vi "Establish connection.vi"(8 "error in (no error)":errorcluster, 11 "TCP Writer in":refnum<class "TCP Writer.lvclass">) -> (0 "error out":errorcluster, 3 "output cluster":refnum<class "TCP Writer.lvclass">)   [LabVIEW 2026, in "TALOS.lvlib" / "TCP Writer.lvlib" / "TCP Writer.lvclass"]
uses:
  TCP Writer.lvclass
  TCP Writer.lvclass/TCP Writer.ctl
  Support VIs/Global Constants.vi
  TALOS.lvlib
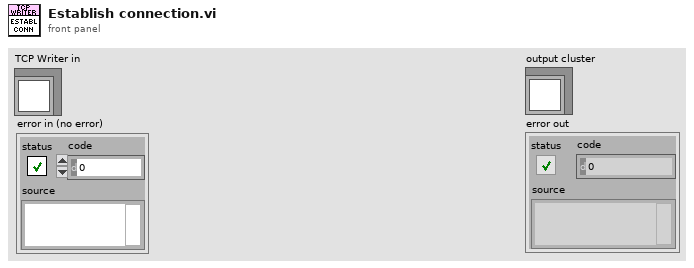
[diagram p1: front panel]
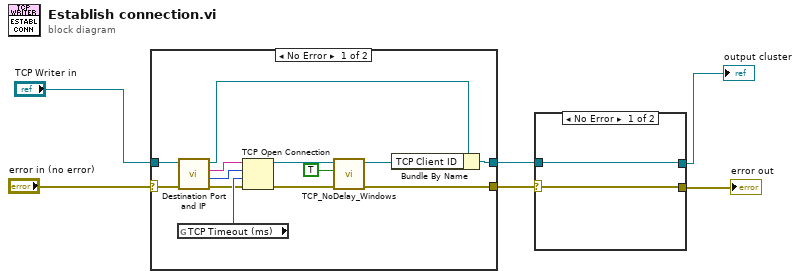
[diagram p0: block diagram]
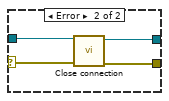
[diagram p3: hidden frame]
diagram:
  n1 = case shown="No Error" "error in (no error)" {
    selector: "error in (no error)" -> [w12 w20]
    tunnel: "TCP Writer in" -> [w14 w21]
    tunnel: [w8 w20] -> w4
    tunnel: [w7 w21] -> w3
    frame No Error {
      n2 = global read "Global Constants.vi" "TCP Timeout (ms)"() -> (w19:i32)
      n3 = call-dynamic "Destination Port and IP.vi"("error in (no error)"=w12, "TCP Writer in"=w14) -> ("error out"=w18:errorcluster, "Destination Port"=w16:u16, "Destination IP"=w17:string, "TCP Writer out"=w13:refnum<class "TCP Writer.lvclass">)  [unwired: 6 in]
      n4 = TCP Open Connection(address=w17, remote port or service name=w16, timeout ms (60000)=w19, error in (no error)=w18) -> (connection ID=w10:refnum<k5>, error out=w11:errorcluster)  [unwired: 1 in]
      n5 = call "TCP_NoDelay_Windows.vi"("error in (no error)"=w11, "TCP_NODELAY (true)"=TRUE, "connID"=w10) -> ("error out"=w8:errorcluster, "connID 2"=w9:refnum<k5>)  [unwired: 3 in]
      n6 = Bundle By Name(cluster=w13, "TCP Client ID"=w9) -> (w7:refnum<class "TCP Writer.lvclass">)
    }
    frame Error {
    }
  }
  n7 = case shown="No Error" w4 {
    selector: w4 -> [w22 w26]
    tunnel: w3 -> [w23 w27]
    tunnel: [w22 w25] -> w2
    tunnel: [w23 w24] -> w1
    frame No Error {
    }
    frame Error {
      n8 = call-dynamic "Close connection.vi"("error in (no error)"=w26, "TCP Writer in"=w27) -> ("error out"=w25:errorcluster, "TCP Writer out"=w24:refnum<class "TCP Writer.lvclass">)  [unwired: 8 in]
    }
  }
  "output cluster" <- w1
  "error out" <- w2
